vi "SignalProcess.vi"(7 "Enabled":bool, 8 "Warning High":dbl, 9 "Warning Low":dbl, 11 "Signal":dbl) -> (0 "Warning":bool, 1 "Disable":i32, 3 "Signal Out":dbl)   [LabVIEW 2016]
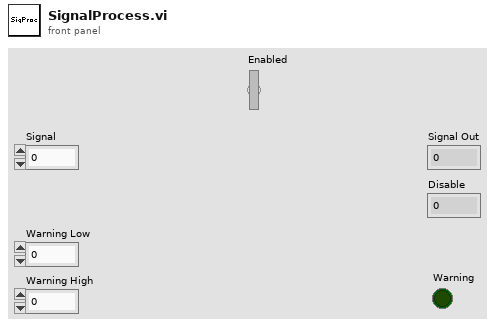
[diagram p1: front panel]
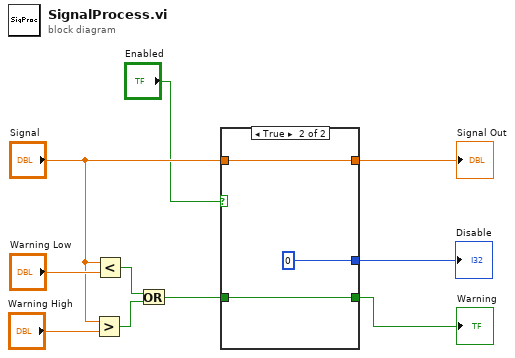
[diagram p0: block diagram]
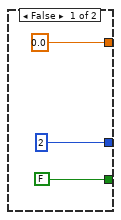
[diagram p2: hidden frame]
diagram:
  n1 = Greater?(x="Signal", y="Warning High") -> (0:w7:bool)
  n2 = Less?(x="Signal", y="Warning Low") -> (x < y?=w8:bool)
  n3 = Or(x=w8, y=w7) -> (x .or. y?=w2:bool)
  n4 = case shown="True" "Enabled" {
    tunnel: [0.0 w16] -> w6
    tunnel: "Signal" -> [_ w16]
    tunnel: [2 0] -> w5
    tunnel: [FALSE w14] -> w3
    tunnel: w2 -> [_ w14]
    frame False {
    }
    frame True {
    }
  }
  "Signal Out" <- w6
  "Warning" <- w3
  "Disable" <- w5
